vi "DSF.Engine.Memory.BufferPool.Set Index FIFO.vi"(8 "error in (no error)":errorcluster, 10 "Index FIFO":refnum<k33>, 11 "BufferPool in":refnum<class "DSF.Engine.Memory.BufferPool.lvclass">) -> (0 "error out":errorcluster, 3 "BufferPool out":refnum<class "DSF.Engine.Memory.BufferPool.lvclass">)   [LabVIEW 2016, in "DSF.Engine.lvlib" / "DSF.Engine.Memory.BufferPool.lvclass"]
uses:
  DSF.Engine.Memory.BufferPool.lvclass
  DSF.Engine.Memory.BufferPool.lvclass/DSF.Engine.Memory.BufferPool.ctl
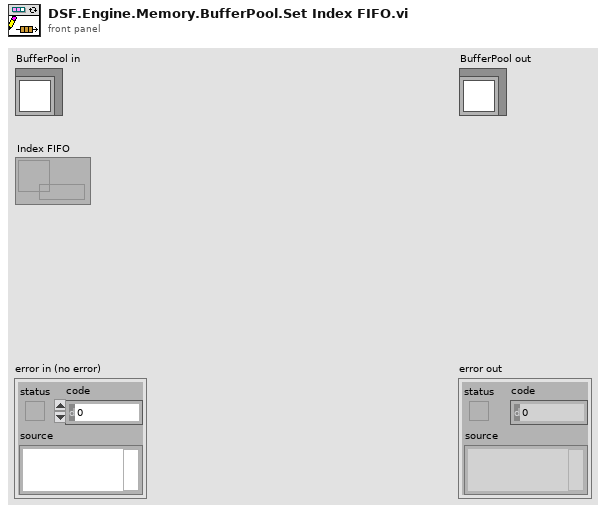
[diagram p1: front panel]
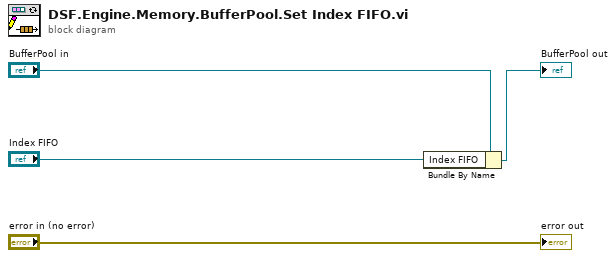
[diagram p0: block diagram]
diagram:
  n1 = Bundle By Name(cluster="BufferPool in", "Index FIFO"="Index FIFO") -> (→"BufferPool out":refnum<class "DSF.Engine.Memory.BufferPool.lvclass">)
  "error out" <- "error in (no error)"
